vi "LED Control.vi"() -> ()   [LabVIEW 2022 SP3]
panel:
  in  "Numeric 2":dbl
  in  "VISA resource name 2":refnum<visa-resource-name>
  out "Connected":bool
  in  "Connect":bool
  in  "Numeric":dbl
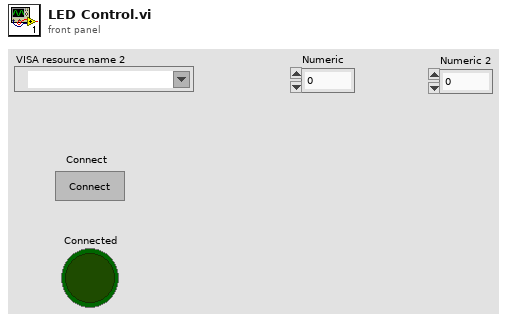
[diagram p1: front panel]
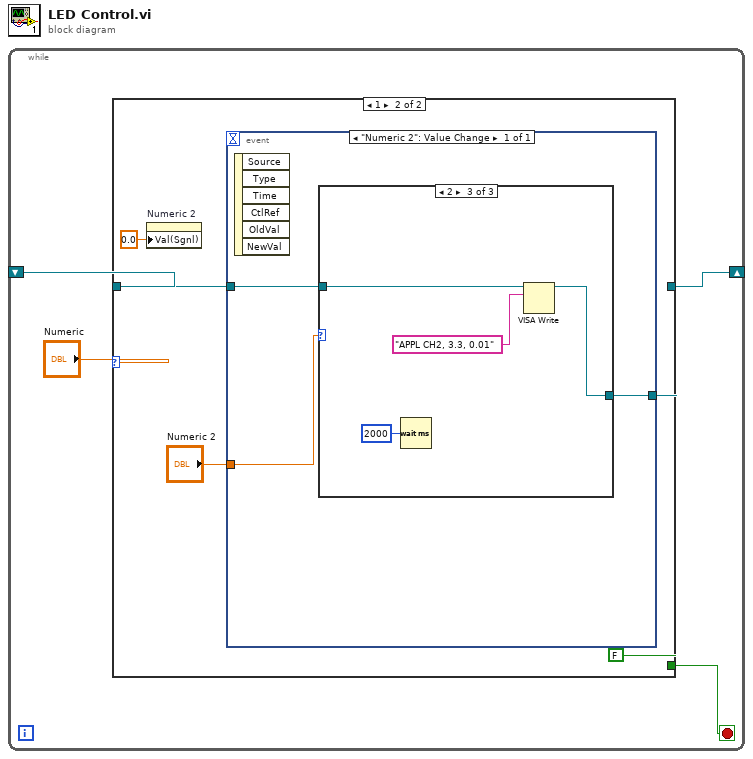
[diagram p0: block diagram]
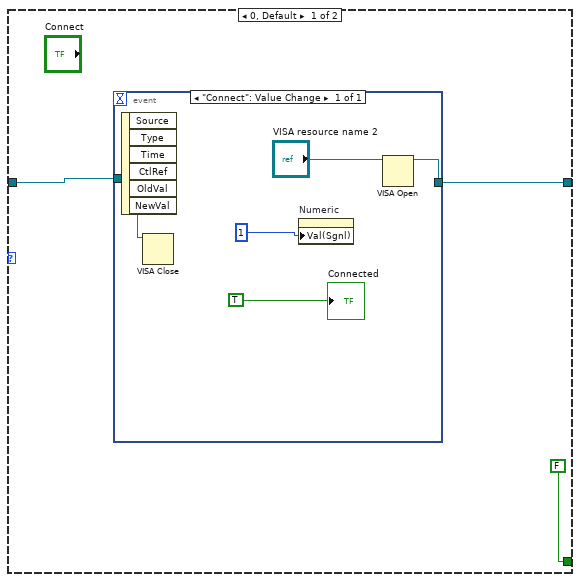
[diagram p2: hidden frame]
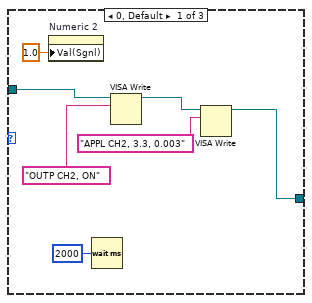
[diagram p3: hidden frame]
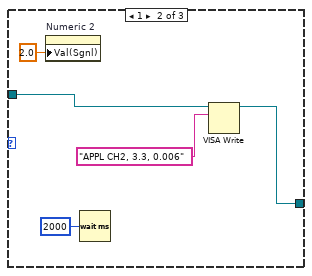
[diagram p4: hidden frame]
diagram:
  n1 = while {
    shift-right: [w3] -> _
    shift-left: _ -> [w4]
    stop <- w1 stop-if-true
    n2 = case shown="1" "Numeric" {
      tunnel: w4 -> [w7 w17]
      tunnel: [w6 w16] -> w3
      tunnel: [FALSE FALSE] -> w1
      frame 0, Default {
        n3 = event shown="[0] \"Connect\": Value Change" {
          selector: _ -> [_]
          dyn-events: _ -> [_]
          timeout: _ -> [_]
          tunnel: [w11] -> w6
          tunnel: w7 -> [w9]
          event "Connect": Value Change {
            n4 = event-data() -> ()  [unwired: 1 in, 6 out]
            n5 = VISA Close(VISA resource name=w9) -> ()  [unwired: 1 in, 1 out]
            n6 = property on="Numeric" class="DigNum (strict)"("Val(Sgnl)"=1) -> ()  [unwired: 2 in, 2 out]
            n7 = VISA Open(VISA resource name="VISA resource name 2") -> (VISA resource name=w11:refnum<visa-resource-name>)  [unwired: 4 in, 1 out]
            "Connected" <- TRUE
          }
        }
      }
      frame 1 {
        n8 = property on="Numeric 2" class="DigNum (strict)"("Val(Sgnl)"=0.0 ("Value (Signaling)")) -> ()  [unwired: 2 in, 2 out]
        n9 = event shown="[0] \"Numeric 2\": Value Change" {
          selector: _ -> [_]
          dyn-events: _ -> [_]
          timeout: _ -> [_]
          tunnel: w17 -> [w20]
          tunnel: [w19] -> w16
          tunnel: "Numeric 2" -> [w18]
          event "Numeric 2": Value Change {
            n10 = event-data() -> ()  [unwired: 1 in, 6 out]
            n11 = case shown="2" w18 {
              tunnel: w20 -> [w23 w28 w33]
              tunnel: [w22 w30 w34] -> w19
              frame 0, Default {
                n12 = property on="Numeric 2" class="DigNum (strict)"("Val(Sgnl)"=1.0 ("Value (Signaling)")) -> ()  [unwired: 2 in, 2 out]
                n13 = Wait (ms)(milliseconds to wait=u32 2000) -> ()  [unwired: 1 out]
                n14 = VISA Write(VISA resource name=w23, write buffer="OUTP CH2, ON") -> (VISA resource name out=w25:refnum<visa-resource-name>)  [unwired: 1 in, 2 out]
                n15 = VISA Write(VISA resource name=w25, write buffer="APPL CH2, 3.3, 0.003") -> (VISA resource name out=w22:refnum<visa-resource-name>)  [unwired: 1 in, 2 out]
              }
              frame 1 {
                n16 = property on="Numeric 2" class="DigNum (strict)"("Val(Sgnl)"=2.0 ("Value (Signaling)")) -> ()  [unwired: 2 in, 2 out]
                n17 = Wait (ms)(milliseconds to wait=u32 2000) -> ()  [unwired: 1 out]
                n18 = VISA Write(VISA resource name=w28, write buffer="APPL CH2, 3.3, 0.006") -> (VISA resource name out=w30:refnum<visa-resource-name>)  [unwired: 1 in, 2 out]
              }
              frame 2 {
                n19 = Wait (ms)(milliseconds to wait=u32 2000) -> ()  [unwired: 1 out]
                n20 = VISA Write(VISA resource name=w33, write buffer="APPL CH2, 3.3, 0.01") -> (VISA resource name out=w34:refnum<visa-resource-name>)  [unwired: 1 in, 2 out]
              }
            }
          }
        }
      }
    }
  }
